vi "View-Buttons.vi"() -> ()   [LabVIEW 2021]
panel:
  in  "tonal--text--rounded":bool
  in  "tonal--text--rectangular":bool
  in  "outline--text--rounded":bool
  in  "outline--text--rectangular":bool
  in  "nooutline--text--rounded":bool
  in  "nooutline--text--rectangular":bool
  in  "filled--text--rounded":bool
  in  "filled--text--rectangular":bool
  in  "tonal--icon--rounded":bool
  in  "tonal--icon--rectangular":bool
  in  "outline--icon--rounded":bool
  in  "outline--icon--rectangular":bool
  in  "nooutline--icon--rounded":bool
  in  "nooutline--icon--rectangular":bool
  in  "filled--icon--rounded":bool
  in  "filled--icon--rectangular":bool
  in  "FAB--icon--rounded":bool
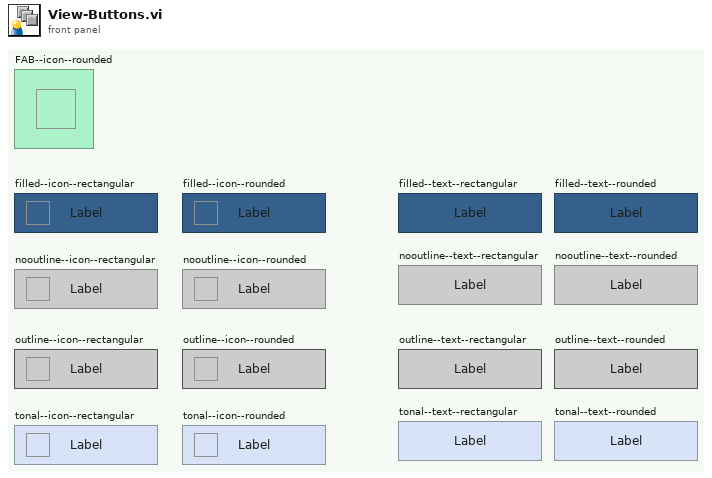
[diagram p1: front panel]
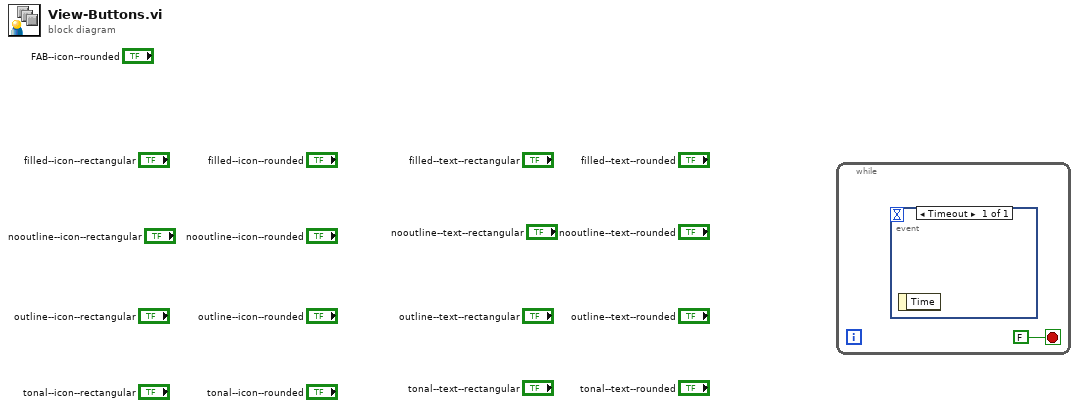
[diagram p0: block diagram]
diagram:
  n1 = while {
    stop <- FALSE stop-if-true
    n2 = event shown="[0] Timeout" {
      selector: _ -> [_]
      dyn-events: _ -> [_]
      timeout: _ -> [_]
      event Timeout {
        n3 = event-data() -> ()  [unwired: 1 in, 1 out]
      }
    }
  }
